vi "Calculate Q0.vi"(8 "error in (no error)":errorcluster, 9 "dt":dbl=1e-06 format="%#_13g", 10 "Data":dbl[][](array[numeric]), 11 "Scope5761 in":refnum<class "Scope5782_six_channel.lvclass">) -> (0 "error out":errorcluster, 1 "Q0 error":bool, 2 "Data out":dbl[][](array[numeric]), 3 "Scope5761out":refnum<class "Scope5782_six_channel.lvclass">)   [LabVIEW 2025, in "Scope5782_six_channel.lvclass"]
uses:
  Scope5782_six_channel.lvclass
  Scope5782_six_channel.lvclass/Scope5782_six_channel.ctl
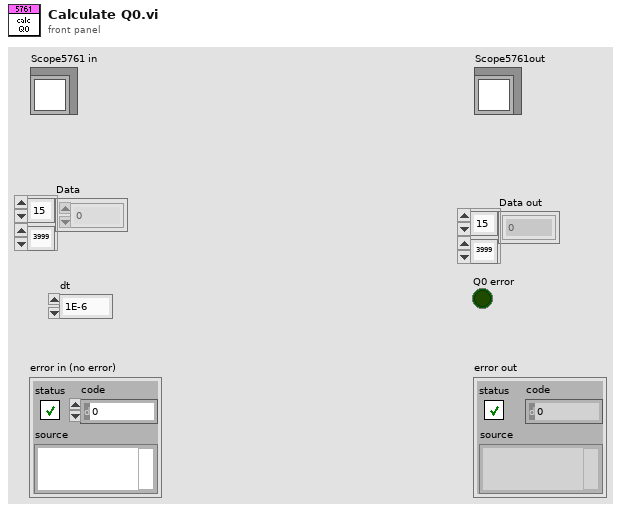
[diagram p1: front panel]
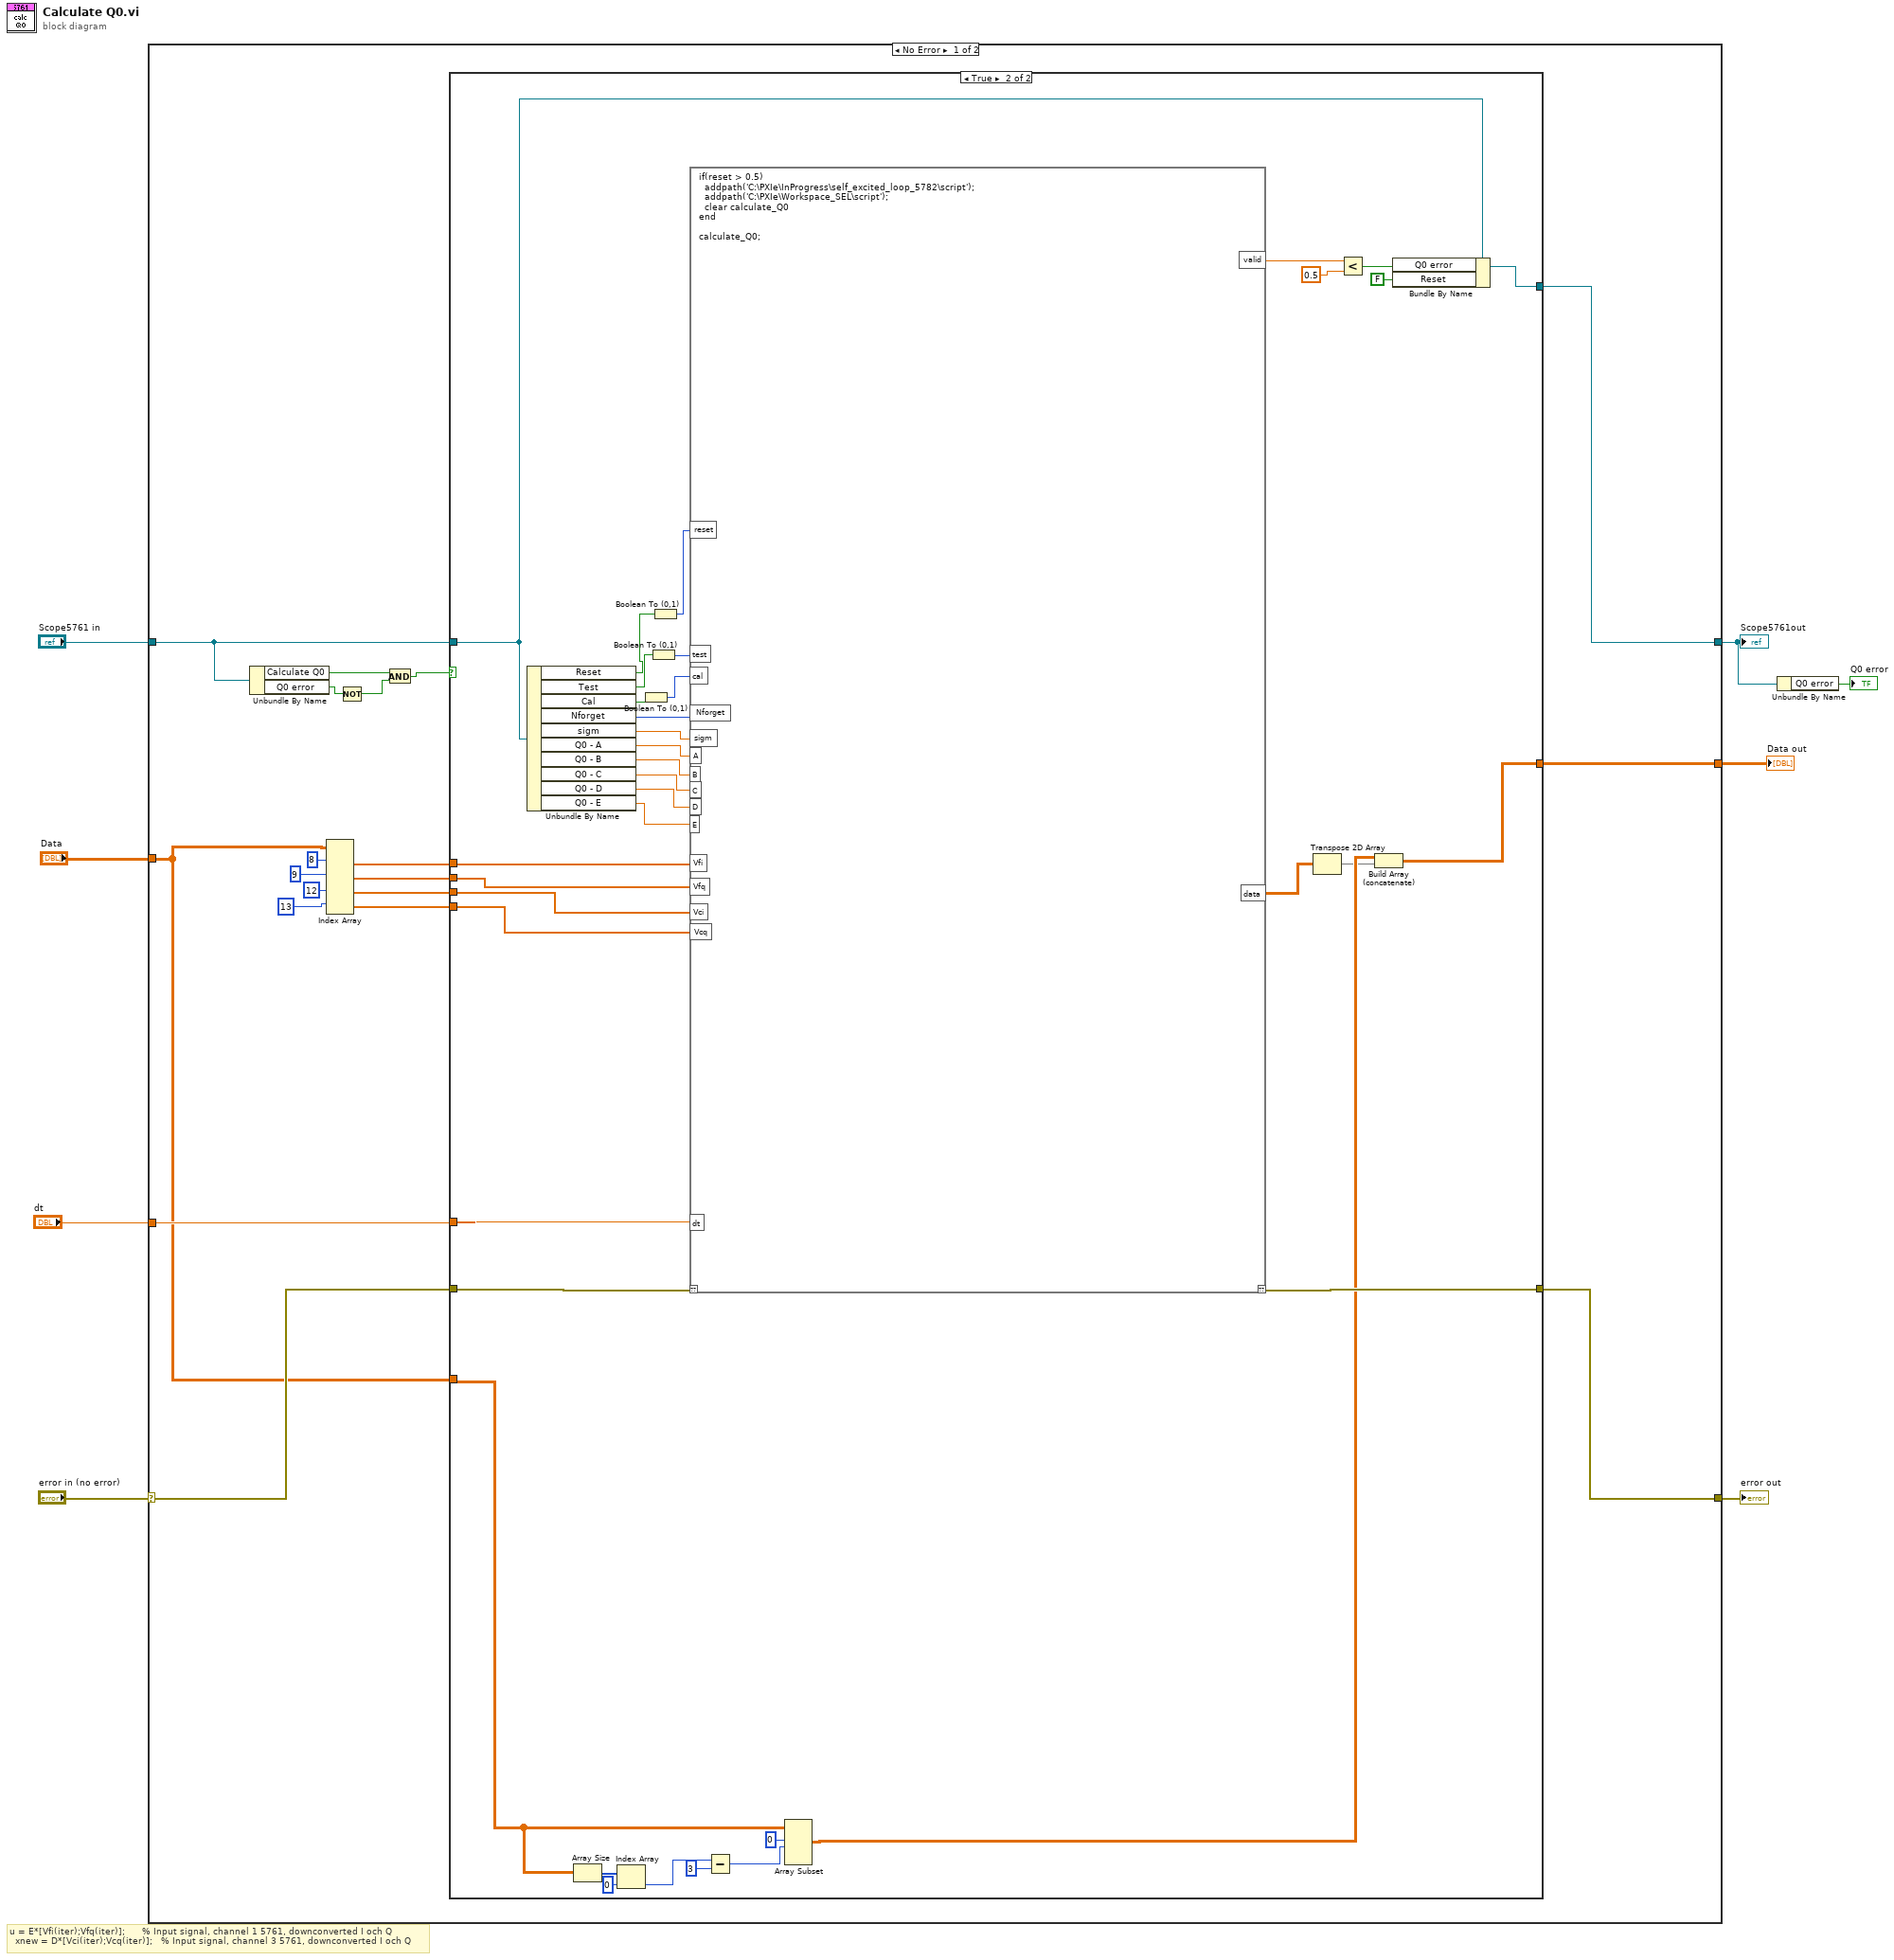
[diagram p0: block diagram]
diagram:
  # "u = E*[Vfi(iter);Vfq(iter)];      % Input signal, channel 1 5761, downconverted I och Q \n  xnew = D*[Vci(iter);Vcq(iter)];   % Input signal, channel 3 5761, downconverted I och Q"
  n1 = case shown="No Error" "error in (no error)" {
    selector: "error in (no error)" -> [w21 w70]
    tunnel: [w20 w70] -> w7
    tunnel: [w9 w69] -> w2
    tunnel: "Scope5761 in" -> [w23 w69]
    tunnel: "Data" -> [w15 w68]
    tunnel: "dt" -> [w22 _]
    tunnel: [w14 w68] -> w3
    frame No Error {
      n2 = Unbundle By Name(w23) -> ("Calculate Q0"=w11:bool, "Q0 error"=w13:bool)
      n3 = Index Array(array=w15, index (row) #1=8 ("index (row)"), index (row) #2=9 ("index (row)"), index (row) #3=12 ("index (row)"), index (row) #4=13 ("index (row)")) -> (element #1=w19:dbl[], element #2=w18:dbl[], element #3=w17:dbl[], element #4=w16:dbl[])  [unwired: 4 in]
      n4 = Not(x=w13) -> (.not. x?=w12:bool)
      n5 = And(x=w11, y=w12) -> (x .and. y?=w10:bool)
      n6 = case shown="True" w10 {
        tunnel: w23 -> [w29 w36]
        tunnel: w22 -> [_ w60]
        tunnel: w21 -> [w30 w59]
        tunnel: [w30 w58] -> w20
        tunnel: w19 -> [_ w57]
        tunnel: w18 -> [_ w56]
        tunnel: w17 -> [_ w55]
        tunnel: w16 -> [_ w54]
        tunnel: [w29 w34] -> w9
        tunnel: w15 -> [w28 w43]
        tunnel: [w28 w45] -> w14
        frame False {
        }
        frame True {
          n7 = Unbundle By Name(w36) -> ("Reset"=w32:bool, "Test"=w42:bool, "Cal"=w40:bool, "Nforget"=w67:i32, "sigm"=w66:dbl, "Q0 - A"=w65:dbl, "Q0 - B"=w64:dbl, "Q0 - C"=w63:dbl, "Q0 - D"=w62:dbl, "Q0 - E"=w61:dbl)
          n8 = Array Size(array=w43) -> (size(s)=w53:i32[])
          n9 = Index Array(array=w53, index=0) -> (element=w51:i32)
          n10 = Boolean To (0,1)(Boolean=w40) -> (0, 1=w39:i16)
          n11 = Boolean To (0,1)(Boolean=w42) -> (0, 1=w41:i16)
          n12 = Boolean To (0,1)(Boolean=w32) -> (0, 1=w33:i16)
          n13 = script code="if(reset > 0.5)\n  addpath('C:\\PXIe\\InProgress\\self_excited_loop_5782\\script');\n  addpath('C:\\PXIe\\Workspace_SEL\\script');\n  clear calculate_Q0\nend\n\ncalculate_Q0;"("??"=w59, "Nforget"=w67, "sigm"=w66, "dt"=w60, "A"=w65, "B"=w64, "C"=w63, "D"=w62, "E"=w61, "Vfi"=w57, "Vfq"=w56, "Vci"=w55, "Vcq"=w54, "test"=w41, "cal"=w39, "reset"=w33) -> ("??"=w58:errorcluster, "data"=w46:dbl[][], "valid"=w38:dbl)
          n14 = Subtract(x=w51, y=3) -> (x-y=w49:i32)
          n15 = Array Subset(array=w43, index (row)=0 ("index"), length (row)=w49) -> (w47:dbl[][])  [unwired: 2 in]
          n16 = Transpose 2D Array(2D array=w46) -> (transposed array=w44:dbl[][])
          n17 = Less?(x=w38, y=0.5) -> (x < y?=w35:bool)
          n18 = Build Array (concatenate)(w47, w44) -> (w45:dbl[][])
          n19 = Bundle By Name(cluster=w36, "Q0 error"=w35, "Reset"=FALSE ("Q0 params.Reset")) -> (w34:refnum<class "Scope5782_six_channel.lvclass">)
        }
      }
    }
    frame Error {
    }
  }
  "error out" <- w7
  "Scope5761out" <- w2
  "Data out" <- w3
  n20 = Unbundle By Name(w2) -> ("Q0 error"=→"Q0 error":bool)
